vi "Profile Status.vi"(8 "error in (no error)":errorcluster, 11 "Temp Chamber in":refnum<class "Temp Chamber.lvclass">) -> (0 "error out":errorcluster, 2 "Status":T1={"Profile Status"={"Profile State"=enum."Not Running", "Current Profile"=0, "Total Time Remaining"=0, "Total Steps"=0}, "Step Status"={"Current Step"=0, "Step Type"=enum."Instant Change", "Time Remaining"=0}}, 3 "Temp Chamber out":refnum<class "Temp Chamber.lvclass">)   [LabVIEW 2018, in "Temp Chamber.lvlib" / "Temp Chamber.lvclass"]
doc: "This Override is used to read a Profile Status."
uses:
  Temp Chamber.lvclass
  Custom Controls/Status.ctl
  Custom Controls/Profile Status.ctl
  Custom Controls/Profile State.ctl
  Custom Controls/Step Status.ctl
  Custom Controls/Step Type.ctl
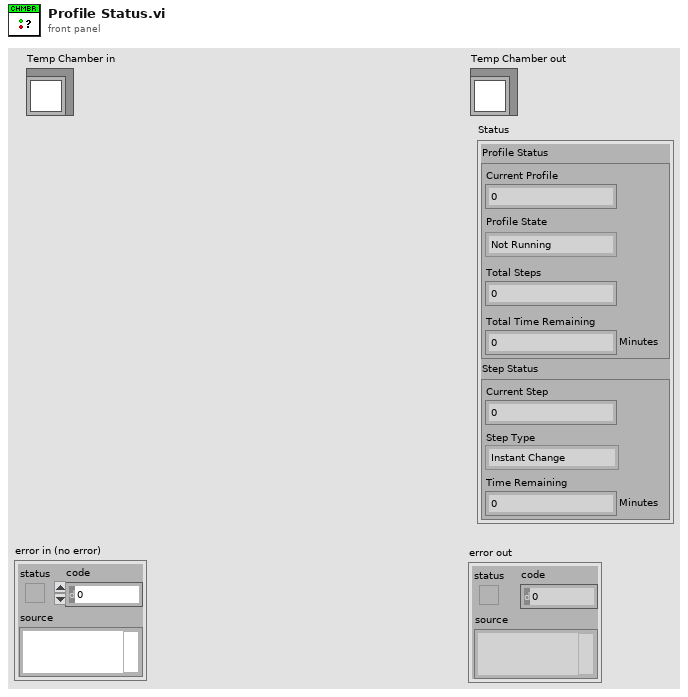
[diagram p1: front panel]
types:
  T1 = typedef "Temp Chamber.lvlib/Temp Chamber.lvclass/Status.ctl" = cluster{"Profile Status":T2, "Step Status":T4}
  T2 = typedef "Temp Chamber.lvlib/Temp Chamber.lvclass/Profile Status.ctl" = cluster{"Profile State":T3, "Current Profile":u32, "Total Time Remaining":u32, "Total Steps":u32}
  T3 = typedef "Temp Chamber.lvlib/Temp Chamber.lvclass/Profile State.ctl" = enum16{"Running", "Not Running", "Paused", "Completed", "Terminated"}
  T4 = typedef "Temp Chamber.lvlib/Temp Chamber.lvclass/Step Status.ctl" = cluster{"Current Step":u32, "Step Type":T5, "Time Remaining":u32}
  T5 = typedef "Temp Chamber.lvlib/Temp Chamber.lvclass/Step Type.ctl" = enum16{"Instant Change", "Wait For", "Jump", "Soak", "Ramp Rate", "Ramp Time", "End", "Other"}
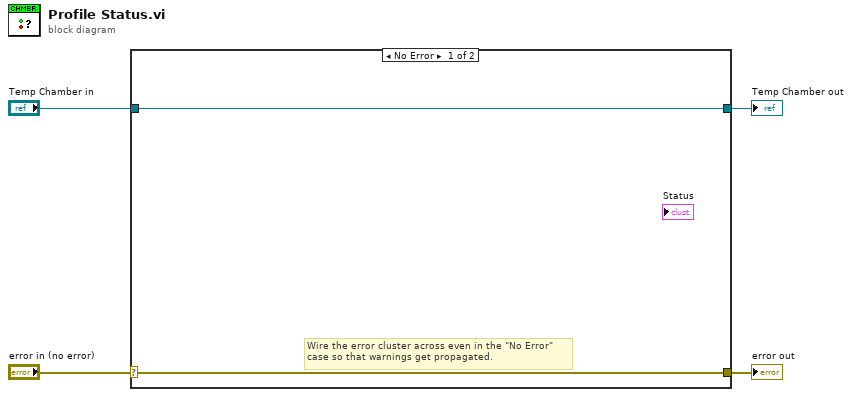
[diagram p0: block diagram]
diagram:
  n1 = case shown="No Error" "error in (no error)" {
    selector: "error in (no error)" -> [w5 w8]
    tunnel: [w5 w8] -> w3
    tunnel: [w6 w7] -> w1
    tunnel: "Temp Chamber in" -> [w6 w7]
    frame No Error {
      # "Wire the error cluster across even in the \"No Error\"\ncase so that warnings get propagated."
    }
    frame Error {
    }
  }
  "error out" <- w3
  "Temp Chamber out" <- w1
